vi "FTW-TestExecutive-Core_Start.vi"(0 "FTW-TestExecutive-Core In":refnum<class "FTW-TestExecutive-Core.lvclass">, 11 "error in":errorcluster) -> (4 "FTW-TestExecutive-Core Out":refnum<class "FTW-TestExecutive-Core.lvclass">, 15 "error out":errorcluster)   [LabVIEW 2015, in "FTW-TestExecutive-Core.lvclass"]
uses:
  FTW-TestExecutive-Core.lvclass
  FTW-TestExecutive-Core.lvclass/FTW-TestExecutive-Core.ctl
  FTW-TestExecutive-Core_State.ctl
  source/actor/Instance/FTW-ActorInstance.lvclass
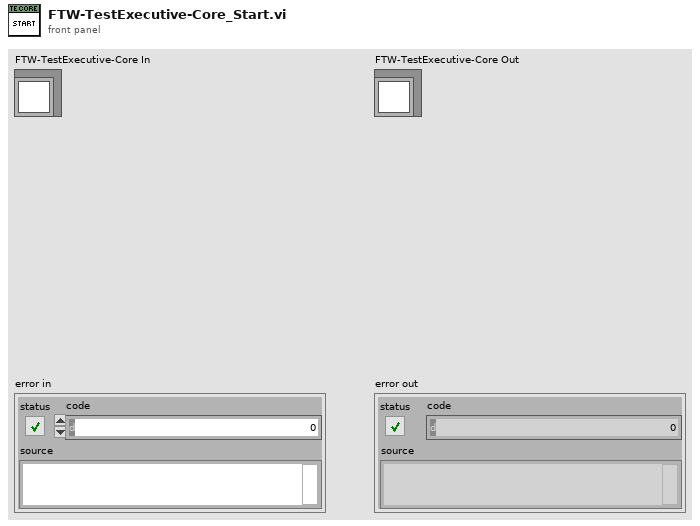
[diagram p1: front panel]
types:
  T1 = typedef "FTW-TestExecutive-Core.lvclass/FTW-TestExecutive-Core_State.ctl" = enum8{"Unloaded", "Loaded", "Executing", "Paused"}
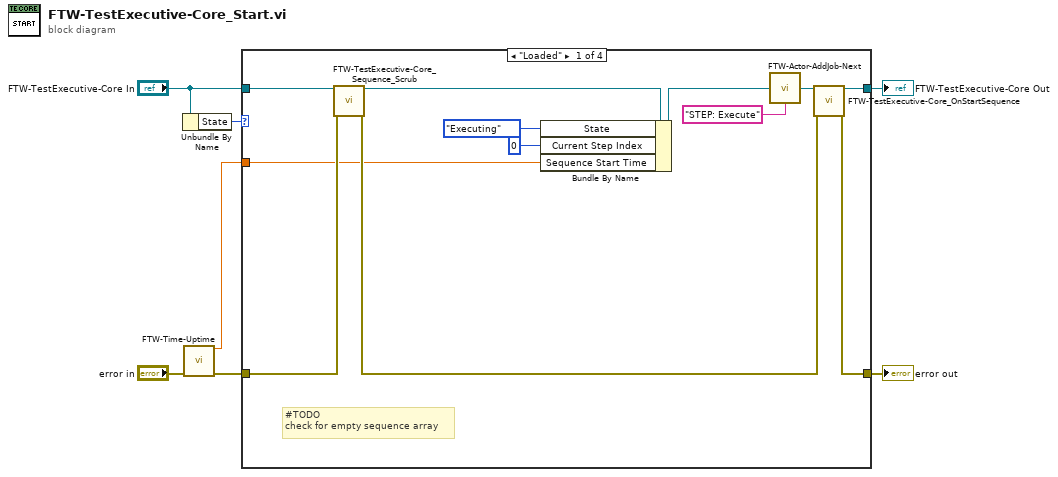
[diagram p0: block diagram]
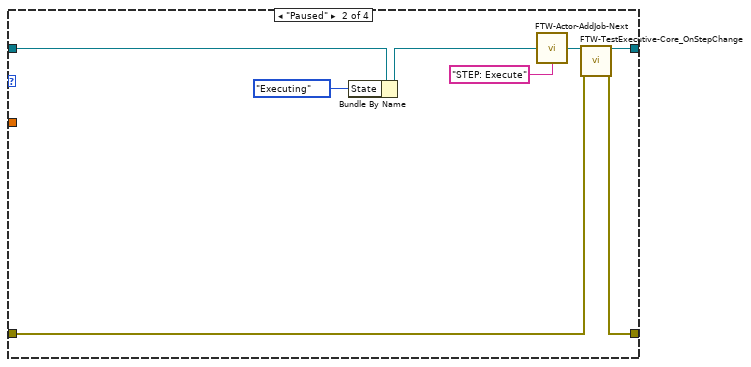
[diagram p2: hidden frame]
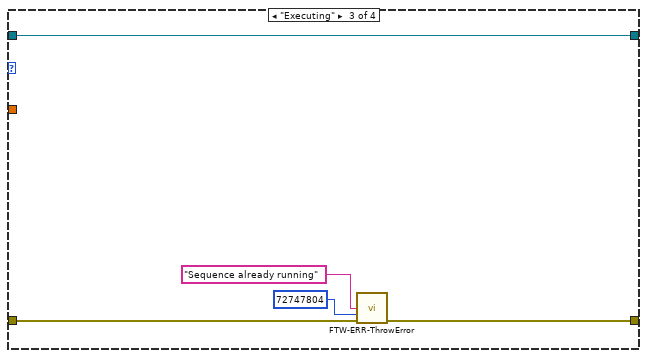
[diagram p3: hidden frame]
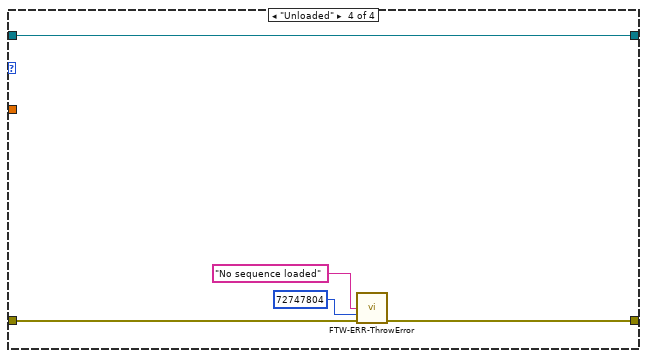
[diagram p4: hidden frame]
diagram:
  n1 = Unbundle By Name("FTW-TestExecutive-Core In") -> ("State"=w5:T1)
  n2 = call "FTW-Time-Uptime.vi"("error in"="error in") -> ("Current Uptime"=w1:dbl, "error out"=w2:errorcluster)  [unwired: 12 in, 1 out]
  n3 = case shown="\"Loaded\"" w5 {
    tunnel: [w13 w22 w32 w37] -> w7
    tunnel: "FTW-TestExecutive-Core In" -> [w17 w25 w32 w37]
    tunnel: [w12 w21 w30 w35] -> w4
    tunnel: w2 -> [w10 w20 w31 w36]
    tunnel: w1 -> [w8 _ _ _]
    frame "Loaded" {
      # "#TODO\ncheck for empty sequence array"
      n4 = call "FTW-TestExecutive-Core_Sequence_Scrub.vi"("FTW-TestExecutive-Core In"=w17, "error in"=w10) -> ("FTW-TestExecutive-Core Out"=w11:refnum<class "FTW-TestExecutive-Core.lvclass">, "error out"=w9:errorcluster)  [unwired: 12 in]
      n5 = Bundle By Name(cluster=w11, "State"=FTW-TestExecutive-Core_State."Executing", "Current Step Index"=0 ("Pointer"), "Sequence Start Time"=w8) -> (w19:refnum<class "FTW-TestExecutive-Core.lvclass">)
      n6 = call "FTW-Actor-AddJob-Next.vi"("Add Next in Job Queue"="STEP: Execute", "FTW Actor Instance"=w19) -> ("FTW Actor Instance out"=w15:refnum<class "FTW-TestExecutive-Core.lvclass">)  [unwired: 2 in]
      n7 = call "FTW-TestExecutive-Core_OnStartSequence.vi"("FTW-TestExecutive-Core In"=w15, "error in"=w9) -> ("FTW-TestExecutive-Core Out"=w13:refnum<class "FTW-TestExecutive-Core.lvclass">, "error out"=w12:errorcluster)  [unwired: 12 in]
    }
    frame "Paused" {
      n8 = Bundle By Name(cluster=w25, "State"=FTW-TestExecutive-Core_State."Executing") -> (w27:refnum<class "FTW-TestExecutive-Core.lvclass">)
      n9 = call "FTW-Actor-AddJob-Next.vi"("Add Next in Job Queue"="STEP: Execute", "FTW Actor Instance"=w27) -> ("FTW Actor Instance out"=w24:refnum<class "FTW-TestExecutive-Core.lvclass">)  [unwired: 2 in]
      n10 = call "FTW-TestExecutive-Core_OnStepChange.vi"("FTW-TestExecutive-Core In"=w24, "error in"=w20) -> ("FTW-TestExecutive-Core Out"=w22:refnum<class "FTW-TestExecutive-Core.lvclass">, "error out"=w21:errorcluster)  [unwired: 12 in]
    }
    frame "Executing" {
      n11 = call "FTW-ERR-ThrowError.vi"("Error Message"="Sequence already running", "Error Code"=72747804, "error in"=w31) -> ("error out"=w30:errorcluster)  [unwired: 12 in]
    }
    frame "Unloaded" {
      n12 = call "FTW-ERR-ThrowError.vi"("Error Message"="No sequence loaded", "Error Code"=72747804, "error in"=w36) -> ("error out"=w35:errorcluster)  [unwired: 12 in]
    }
  }
  "FTW-TestExecutive-Core Out" <- w7
  "error out" <- w4
